vi "PalmSense State.vi"(7 "Channels":string[](array[combo])=["3", "4"], 8 "error in (no error)":errorcluster, 9 "State":bool, 11 "PS in":refnum<queue>) -> (0 "error out":errorcluster, 3 "PS out":refnum<queue>)   [LabVIEW 2020, in "PalmSens.lvlib"]
uses:
  PalmSens.lvlib
  support/Message Queue/Message Queue.lvlib
  support/Message Queue/Message Cluster.ctl
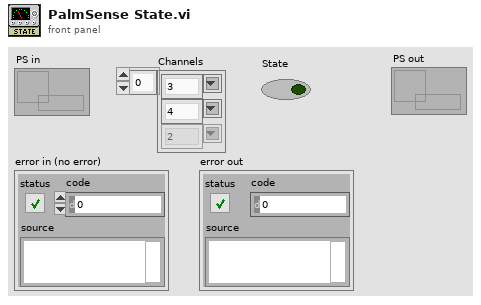
[diagram p1: front panel]
types:
  T1 = cluster{"Channel Name":string, "Enable Output":bool, "Send Resp":bool}
  T2 = cluster{"Type CMD":string, "Mode CMD":string, "Main CMD":string}
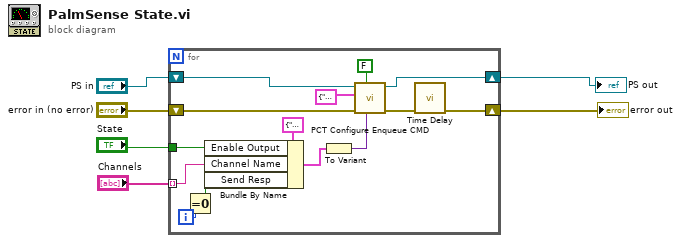
[diagram p0: block diagram]
diagram:
  n1 = for {
    tunnel: "State" -> [w13]
    tunnel: "Channels" -> [w12] mode=indexing
    shift-right: [w10] -> w1
    shift-left: "error in (no error)" -> [w20]
    shift-right: [w14] -> w4
    shift-left: "PS in" -> [w19]
    i -> [w8]
    n2 = Equal To 0?(x=w8) -> (x = 0?=w7:bool)
    n3 = Bundle By Name(cluster=T1 {"Channel Name"="", "Enable Output"=FALSE, "Send Resp"=FALSE}, "Enable Output"=w13, "Channel Name"=w12, "Send Resp"=w7) -> (w15:T1)
    n4 = To Variant(anything=w15) -> (Variant=w17:variant)
    n5 = call "PCT Configure Enqueue CMD.vi"("Parameter Data"=w17, "Read"=FALSE, "error in (no error)"=w20, "CMD"=T2 {"Type CMD"="Output Enabled", "Mode CMD"="", "Main CMD"="Configure"}, "CMD Queue in"=w19) -> ("error out"=w11:errorcluster, "CMD Queue out"=w14:refnum<queue>)  [unwired: 4 in, 1 out]
    n6 = call "Time Delay"("error in (no error)"=w11) -> ("error out"=w10:errorcluster)  [unwired: 10 in]
  }
  "error out" <- w1
  "PS out" <- w4
